vi "SD-Strip Path__ogtk.vi"   [LabVIEW 2020, in "SD-openg_file.lvlib"]
doc: "Functions identically to LabVIEW \"Strip Path\" function, but is polymorphic to also allow the path input to be an array. If an array is used, the outputs become arrays."
uses:
  SD-openg_file.lvlib
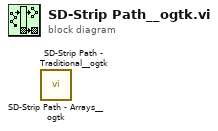
[diagram p0: block diagram]
diagram:
  n1 = call "SD-Strip Path - Arrays__ogtk.vi"() -> ()  [unwired: 1 in, 2 out]
  n2 = call "SD-Strip Path - Traditional__ogtk.vi"() -> ()  [unwired: 1 in, 2 out]
